vi "ICPCON Data Acquisition Loop - FCXF.vi"(7 "sampling period (s)":dbl caption="采用周期 (s)", 8 "error in (no error)":errorcluster caption="错误输入（无错误）", 11 "Message Queues":T1 caption="消息队列") -> (0 "error out":errorcluster caption="错误输出")   [LabVIEW 2015]
uses:
  Support VIs/Message Queue/All Real-Time Message Queues.ctl
  Support VIs/Message Queue/Message Cluster.ctl
  <vilib>/Platform/TimedLoop/XDataNode/timing_clust.ctl
  <vilib>/Platform/TimedLoop/XDataNode/nitl_modes.ctl
  <vilib>/Platform/TimedLoop/XDataNode/wakeup.ctl
  <vilib>/Instr/_visa.llb/VISA Configure Serial Port (Instr).vi
  Globals/Global - Monitoring Variables.vi
  <vilib>/Platform/TimedLoop/XDataNode/loadnilvce.vi
  Globals/Global - All RT Loop Stop.vi
  <vilib>/Platform/TimedLoop/XDataNode/XDataNode.xnode
  <vilib>/Platform/TimedLoop/XDataNode/XDNodeRunTimeDep.lvlib
  Support VIs/Message Queue/Message Queue.lvlib
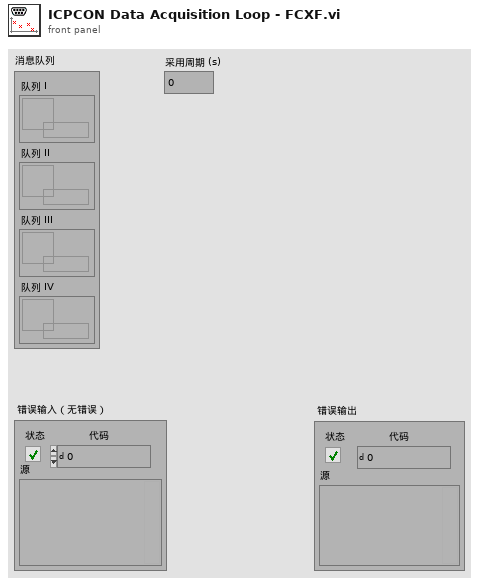
[diagram p1: front panel]
types:
  T1 = typedef "Message Queue.lvlib/All Real-Time Message Queues.ctl" = cluster{"Queue I":refnum<queue>, "Queue II":refnum<queue>, "Queue III":refnum<queue>, "Queue IV":refnum<queue>}
  T2 = typedef "XDNodeRunTimeDep.lvlib/timing_clust.ctl" = cluster{"Expected End [f-1]":u64, "Actual End [f-1]":u64, "Finished Late? [f-1]":bool, "Expected End [i-1]":u64, "Actual End [i-1]":u64, "Finished Late? [i-1]":bool, "Expected Start [i]":u64, "Actual Start [i]":u64, "Expected Start [f]":u64, "Actual Start [f]":u64, "Source Name":string, "Structure Name":string, "Period":i64, "Deadline":i64, "Offset":i64, "Start":i64, "Priority":i32, "Timeout":i32, "Mode":T3, "Wakeup Reason":T4, "Error":errorcluster, "Source Type":string, "Secondary Source Type":string, "Global End Time":u64, "Global Start Time":u64, "Frame Duration":u64, "Iteration Duration":u64, "Assigned CPU":i32, "I/O Scan Engine Mode":u32}
  T3 = typedef "XDNodeRunTimeDep.lvlib/nitl_modes.ctl" = enum32{"No Change", "Process missed periods, maintain original phase", "Discard missed periods, maintain original phase", "Process missed periods, ignore original phase", "Discard missed periods, ignore original phase"}
  T4 = typedef "XDNodeRunTimeDep.lvlib/wakeup.ctl" = enum32{"Normal", "Aborted", "Asynchronous wakeup", "Timing source error", "Timed loop error", "Timeout"}
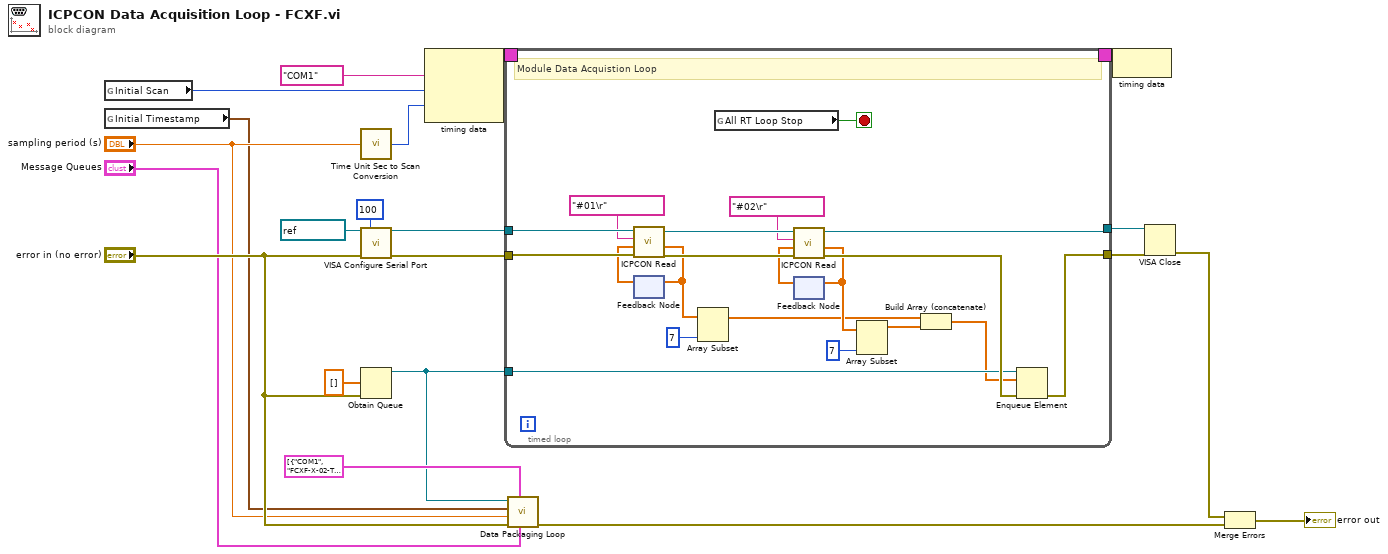
[diagram p0: block diagram]
diagram:
  n1 = global read "Global - Monitoring Variables.vi" "Initial Scan"() -> (w9:i64)
  n2 = global read "Global - Monitoring Variables.vi" "Initial Timestamp"() -> (w1:timestamp)
  n3 = call "Time Unit Sec to Scan Conversion.vi"("time duration (s)"="sampling period (s)") -> ("time duration (scan)"=w8:i64)
  n4 = call-poly "VISA Configure Serial Port"("VISA resource name"=refnum<visa-resource-name> "COM1", "timeout (10sec)"=u32 100, "error in (no error)"="error in (no error)") -> ("VISA resource name out"=w14:refnum<visa-resource-name>, "error out"=w2:errorcluster)  [unwired: 11 in]
  n5 = Obtain Queue(element data type=dbl[] [] ("数据类型"), error in (no error)="error in (no error)") -> (queue out=w5:refnum<queue>)  [unwired: 3 in, 2 out]
  n6 = node-c288("COM1" ("Structure Name"), w9, w8) -> (w20:T2)
  n7 = timed-loop {
    timing: w20 -> [_]
    timing-out: [_] -> w19
    tunnel: w5 -> [w27]
    tunnel: w2 -> [w39]
    tunnel: [w40] -> w16
    tunnel: [w34] -> w17
    tunnel: w14 -> [w38]
    stop <- w41 stop-if-true
    # "Module Data Acquistion Loop"
    n8 = feedback #1() -> (w37:dbl[])  [unwired: 1 in]
    n9 = call "ICPCON Read.vi"("error in (no error)"=w39, "Last Data Array"=w37, "write buffer"="#01\r", "VISA Ref Input"=w38) -> ("error out"=w33:errorcluster, "New Data Array"=w30:dbl[], "VISA Ref Output"=w36:refnum<visa-resource-name>)  [unwired: 5 in]
    n10 = feedback-in #1(w30) -> ()
    n11 = Array Subset(array=w30, length=7 ("长度")) -> (w22:dbl[])  [unwired: 1 in]
    n12 = global read "Global - All RT Loop Stop.vi" "All RT Loop Stop"() -> (w41:bool)
    n13 = feedback #2() -> (w32:dbl[])  [unwired: 1 in]
    n14 = call "ICPCON Read.vi"("error in (no error)"=w33, "Last Data Array"=w32, "write buffer"="#02\r", "VISA Ref Input"=w36) -> ("error out"=w31:errorcluster, "New Data Array"=w29:dbl[], "VISA Ref Output"=w34:refnum<visa-resource-name>)  [unwired: 5 in]
    n15 = feedback-in #2(w29) -> ()
    n16 = Array Subset(array=w29, length=7 ("长度")) -> (w24:dbl[])  [unwired: 1 in]
    n17 = Build Array (concatenate)(w22, w24) -> (w26:dbl[])
    n18 = Enqueue Element(queue=w27, element=w26, error in (no error)=w31) -> (error out=w40:errorcluster)  [unwired: 1 in, 2 out]
  }
  n19 = call "Data Packaging Loop.vi"("Message Queues"="Message Queues", "channel info array"=cluster{"Module":string, "Channel":string}[] [{"Module"="COM1", "Channel"="FCXF-X-02-T01"}, {"Module"="COM1", "Channel"="FCXF-X-02-T02"}, {"Module"="COM1", "Channel"="FCXF-X-02-T03"}, {"Module"="COM1", "Channel"="FCXF-X-02-T04"}, {"Module"="COM1", "Channel"="FCXF-X-03-T01"}, {"Module"="COM1", "Channel"="FCXF-X-03-T02"}, {"Module"="COM1", "Channel"="FCXF-X-03-T03"}, {"Module"="COM1", "Channel"="FCXF-X-03-T04"}, {"Module"="COM1", "Channel"="FCXF-X-03-T05"}, {"Module"="COM1", "Channel"="FCXF-X-03-T06"}, {"Module"="COM1", "Channel"="FCXF-X-04-T01"}, {"Module"="COM1", "Channel"="FCXF-X-04-T02"}, {"Module"="COM1", "Channel"="FCXF-X-04-T03"}, {"Module"="COM1", "Channel"="FCXF-X-04-T04"}], "error in (no error)"="error in (no error)", "sampling period (s)"="sampling period (s)", "timestamp"=w1, "data queue"=w5) -> ("error out"=w6:errorcluster)  [unwired: 5 in]
  n20 = node-c288(w19) -> ()
  n21 = VISA Close(VISA resource name=w17, error in (no error)=w16) -> (error out=w15:errorcluster)
  n22 = Merge Errors(w15, w6) -> (→"error out":errorcluster)
